vi "FM_modulace.vi"(4 "Noise STD":dbl format="%.2p", 6 "Sampling info":cluster{"Fs":dbl, "#s":dbl}={"Fs"=1000.0, "#s"=10000.0}, 7 "Typ signalu nosna":T1(ring), 8 "error in":errorcluster, 9 "Nosna Frekvence (Hz)":dbl=20.0 min=86453.20197044335, 10 "Frekvencni zdvih (Hz)":dbl=8.0, 11 "Modulacni Frekvence (Hz)":dbl=2.0) -> (0 "error out":errorcluster, 1 "Modulacni signal":waveform(dbl)={"t0"=timestamp(0 s since 1904-01-01), "dt"=0.001, "Y"=array[10000 elements]}, 2 "Nosna signal":waveform(dbl)={"t0"=timestamp(0 s since 1904-01-01), "dt"=0.001, "Y"=array[10000 elements]}, 3 "Modulovany signal":waveform(dbl)={"t0"=timestamp(0 s since 1904-01-01), "dt"=0.001, "Y"=array[10000 elements]})   [LabVIEW 2021]
doc: "This example demonstrates how to simulate a Frequency Modulation (FM) using the signal generation functions. This VI also presents the Power Spectrum of the FM signal."
uses:
  <vilib>/measure/maspectr.llb/FFT Power Spectrum and PSD for 1 Chan.vi
  <vilib>/measure/NI_MABase.lvlib
  <vilib>/measure/NI_MAPro.lvlib
panel:
  out "Baseband Graph":waveform(dbl)(graph)={"t0"=timestamp(0 s since 1904-01-01), "dt"=0.001, "Y"=array[10000 elements]}
  out "Carrier Graph":waveform(dbl)(graph)={"t0"=timestamp(0 s since 1904-01-01), "dt"=0.001, "Y"=array[10000 elements]}
  out "Power Spectrum":cluster{"f0":dbl, "df":dbl, "magnitude":dbl[]}(graph)={"f0"=0.0, "df"=0.1, "magnitude"=array[5000 elements]}
  out "Original and modulated":waveform(dbl)[](graph)=[{"t0"=timestamp(0 s since 1904-01-01), "dt"=0.001, "Y"=array[10000 elements]}, {"t0"=timestamp(0 s since 1904-01-01), "dt"=0.001, "Y"=array[10000 elements]}]
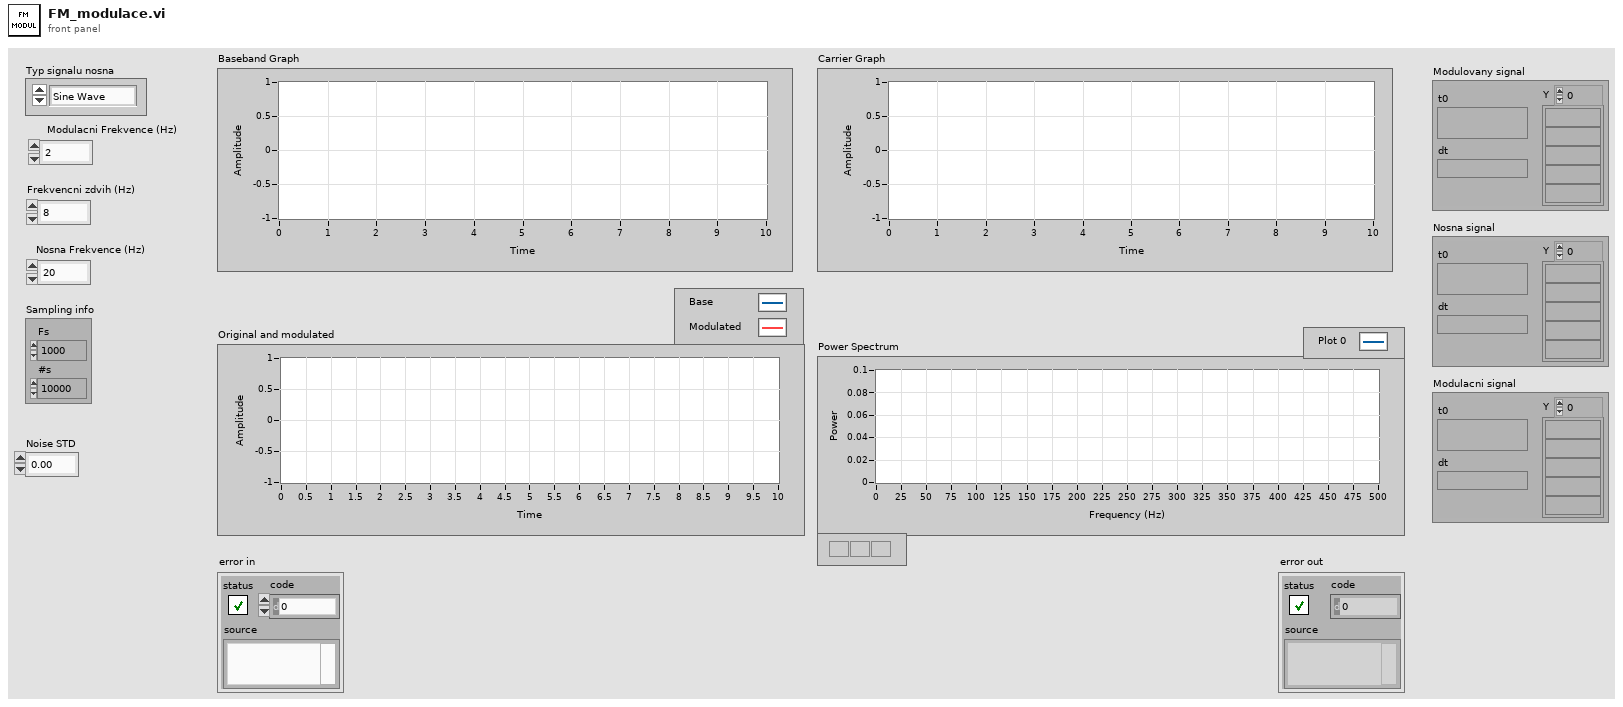
[diagram p1: front panel]
types:
  T1 = enum16{"Sine Wave", "Triangle Wave", "Square Wave", "Sawtooth Wave"}
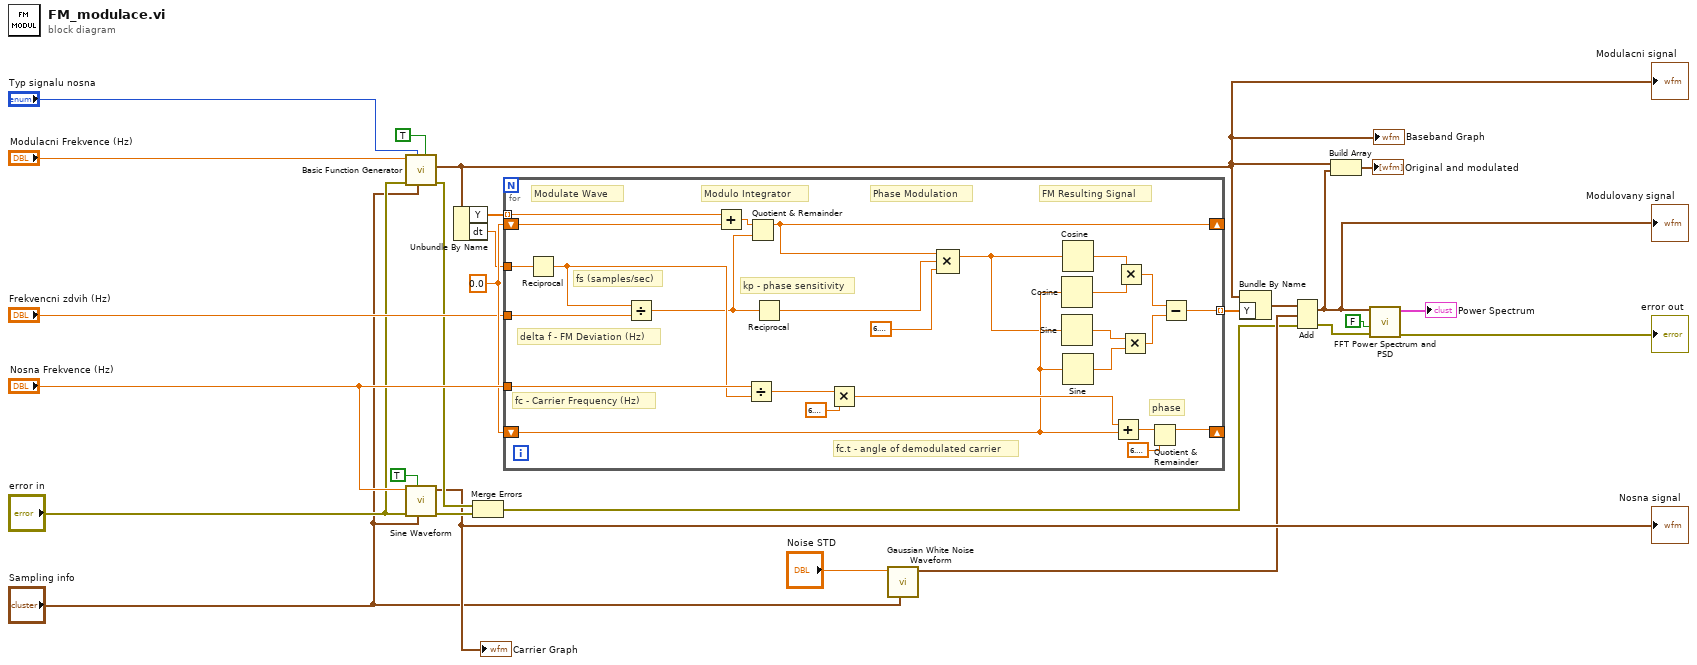
[diagram p0: block diagram]
diagram:
  w23 = 0.0
  n1 = call <vilib>:"Basic Function Generator.vi"("reset signal"=TRUE, "sampling info"="Sampling info", "signal type"="Typ signalu nosna", "error in (no error)"="error in", "frequency"="Modulacni Frekvence (Hz)") -> ("error out"=w11:errorcluster, "signal out"=w7:waveform(dbl))  [unwired: 4 in, 1 out]
  "Baseband Graph" <- w7
  "Modulacni signal" <- w7
  n2 = call <vilib>:"Sine Waveform.vi"("sampling info"="Sampling info", "reset signal"=TRUE, "error in (no error)"="error in", "frequency"="Nosna Frekvence (Hz)") -> ("error out"=w12:errorcluster, "signal out"=→"Carrier Graph" →"Nosna signal":waveform(dbl))  [unwired: 6 in]
  n3 = Unbundle By Name(w7) -> ("Y"=w17:dbl[], "dt"=w20:dbl)
  n4 = Merge Errors(w11, w12) -> (w2:errorcluster)
  n5 = for {
    tunnel: w20 -> [w52]
    tunnel: "Frekvencni zdvih (Hz)" -> [w51]
    shift-right: [w38] -> _
    shift-left: w23 -> [w37]
    tunnel: w17 -> [w36] mode=indexing
    tunnel: "Nosna Frekvence (Hz)" -> [w50]
    tunnel: [w45] -> w19 mode=indexing
    shift-right: [w41] -> _
    shift-left: w23 -> [w34]
    # "fc.t - angle of demodulated carrier"
    # "Modulate Wave"
    # "fc - Carrier Frequency (Hz)"
    # "delta f - FM Deviation (Hz)"
    # "phase"
    # "FM Resulting Signal"
    # "Phase Modulation"
    # "kp - phase sensitivity"
    # "Modulo Integrator"
    # "fs (samples/sec)"
    n6 = Reciprocal(x=w52) -> (1/x=w49:dbl)
    n7 = Divide(x=w49, y=w51) -> (x/y=w39:dbl)
    n8 = Add(x=w36, y=w37) -> (x+y=w40:dbl)
    n9 = Divide(x=w50, y=w49) -> (x/y=w47:dbl)
    n10 = Quotient & Remainder(x=w40, y=w39) -> (x-y*floor(x/y)=w38:dbl)  [unwired: 1 out]
    n11 = Reciprocal(x=w39) -> (1/x=w28:dbl)
    n12 = Multiply(x=w47, y=6.283185307179586) -> (x*y=w44:dbl)
    n13 = Compound Arithmetic op=MULTIPLY(w38, w28, 6.283185307179586) -> (w29:dbl)
    n14 = Cosine(x=w34) -> (cos(x)=w31:dbl)
    n15 = Sine(x=w29) -> (sin(x)=w30:dbl)
    n16 = Cosine(x=w29) -> (cos(x)=w32:dbl)
    n17 = Sine(x=w34) -> (sin(x)=w33:dbl)
    n18 = Add(x=w44, y=w34) -> (x+y=w43:dbl)
    n19 = Multiply(x=w32, y=w31) -> (x*y=w46:dbl)
    n20 = Multiply(x=w30, y=w33) -> (x*y=w35:dbl)
    n21 = Quotient & Remainder(x=w43, y=6.283185307179586) -> (x-y*floor(x/y)=w41:dbl)  [unwired: 1 out]
    n22 = Subtract(x=w46, y=w35) -> (x-y=w45:dbl)
  }
  n23 = call <vilib>:"Gaussian White Noise Waveform.vi"("sampling info"="Sampling info", "standard deviation"="Noise STD") -> ("signal out"=w3:waveform(dbl))  [unwired: 8 in, 1 out]
  n24 = Bundle By Name(cluster=w7, "Y"=w19) -> (w14:waveform(dbl))
  n25 = Add(1:w3, 2:w14, 4:w2) -> (0:w4:waveform(dbl), 3:w1:errorcluster)
  "Modulovany signal" <- w4
  n26 = Build Array(w7, w4) -> (→"Original and modulated":waveform(dbl)[])
  n27 = call-poly <vilib>:"FFT Power Spectrum and PSD.vi"("error in (no error)"=w1, "dB On (F)"=FALSE, "time signal"=w4) -> ("error out"=→"error out":errorcluster, "Power Spectrum / PSD"=→"Power Spectrum":cluster{"f0":dbl, "df":dbl, "magnitude":dbl[]})  [unwired: 5 in, 2 out]
